vi "Cache.Result.Move.vi"(6 "Time (now)":timestamp, 8 "error in":errorcluster, 11 "File":path) -> (0 "error out":errorcluster)   [LabVIEW 2016]
uses:
  Global/ApplicationGlobal.vi
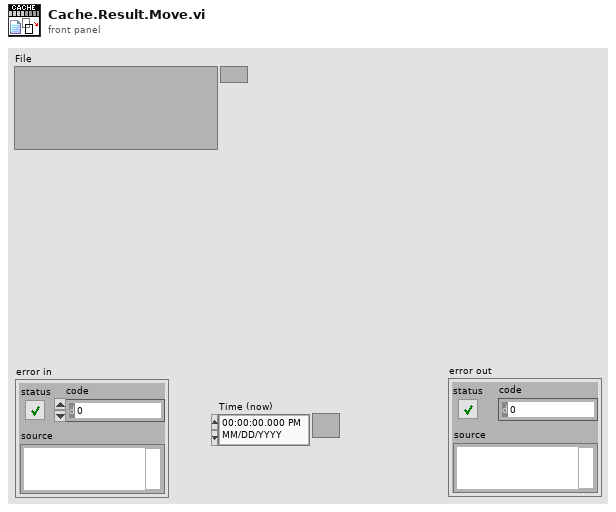
[diagram p1: front panel]
types:
  T1 = enum16{"open", "open or create", "create or replace", "create", "open (read-only)"}
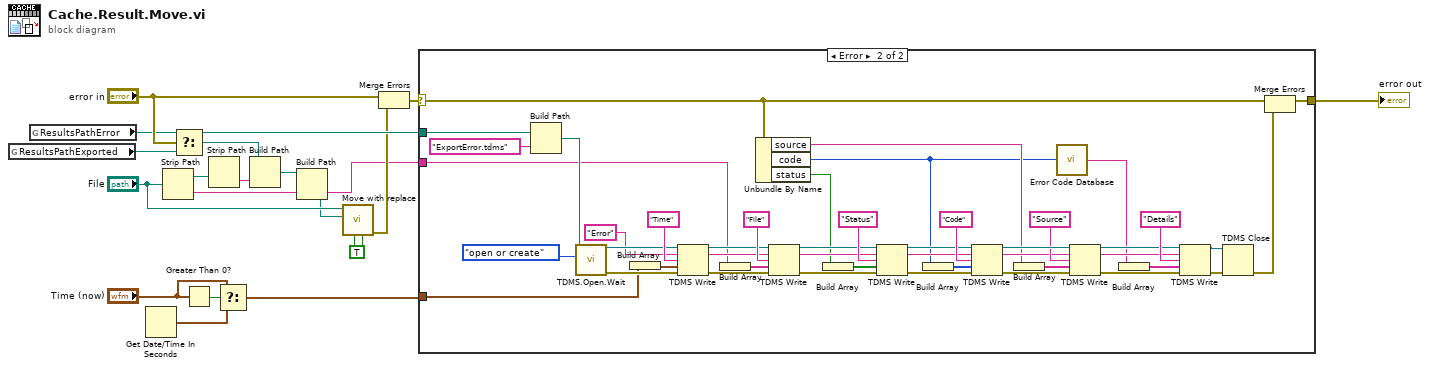
[diagram p0: block diagram]
diagram:
  w1 = TRUE ("create parent dirs (F)")
  n1 = global read "ApplicationGlobal.vi" "ResultsPathExported"() -> (w18:path)
  n2 = global read "ApplicationGlobal.vi" "ResultsPathError"() -> (w16:path)
  n3 = Get Date/Time In Seconds() -> (seconds since 1Jan1904=w12:timestamp)
  n4 = Strip Path(path="File") -> (stripped path=w4:path, name=w6:string)
  n5 = Select(t=w16, s="error in", f=w18) -> (s? t:f=w5:path)
  n6 = Greater Than 0?(x="Time (now)") -> (x > 0?=w13:bool)
  n7 = Strip Path(path=w4) -> (name=w3:string)  [unwired: 1 out]
  n8 = Select(t="Time (now)", s=w13, f=w12) -> (s? t:f=w10:timestamp)
  n9 = Build Path(base path=w5, name or relative path=w3) -> (appended path=w2:path)
  n10 = Build Path(base path=w2, name or relative path=w6) -> (appended path=w8:path)
  n11 = call "Move with replace.vi"("create parent dirs (F)"=w1, "replace allowed (T)"=w1, "destination path"=w8, "source path"="File") -> ("error"=w7:errorcluster)  [unwired: 7 in]
  n12 = Merge Errors("error in", w7) -> (w15:errorcluster)
  n13 = case shown="Error" w15 {
    selector: w15 -> [w19 w22]
    tunnel: w6 -> [_ w30]
    tunnel: w10 -> [_ w20]
    tunnel: w16 -> [_ w52]
    tunnel: [w19 w23] -> w14
    frame No Error {
    }
    frame Error {
      n14 = Build Path(base path=w52, name or relative path="ExportError.tdms") -> (appended path=w50:path)
      n15 = call "TDMS.Open.Wait.vi"("operation (open read-only)"=T1."open or create", "file path"=w50) -> ("error out"=w44:errorcluster, "tdms file out"=w47:refnum<k34>)  [unwired: 8 in]
      n16 = Build Array(w20) -> (w43:timestamp[])
      n17 = TDMS Write(0:w47, 5:"Error" ("group name in (Untitled)"), 7:"Time" ("channel name"), 9:w43, 11:w44) -> (4:w46:refnum<k34>, 6:w37:string, 15:w45:errorcluster)  [unwired: 1 in, 1 out]
      n18 = Build Array(w30) -> (w42:string[])
      n19 = Unbundle By Name(w22) -> ("source"=w28:string, "code"=w27:i32, "status"=w29:bool)
      n20 = TDMS Write(0:w46, 5:w37, 7:"File" ("channel name"), 9:w42, 11:w45) -> (4:w53:refnum<k34>, 6:w40:string, 15:w49:errorcluster)  [unwired: 1 in, 1 out]
      n21 = Build Array(w29) -> (w63:bool[])
      n22 = TDMS Write(0:w53, 5:w40, 7:"Status" ("channel name"), 9:w63, 11:w49) -> (4:w60:refnum<k34>, 6:w39:string, 15:w59:errorcluster)  [unwired: 1 in, 1 out]
      n23 = Build Array(w27) -> (w58:i32[])
      n24 = TDMS Write(0:w60, 5:w39, 7:"Code" ("channel name"), 9:w58, 11:w59) -> (4:w57:refnum<k34>, 6:w38:string, 15:w56:errorcluster)  [unwired: 1 in, 1 out]
      n25 = Build Array(w28) -> (w41:string[])
      n26 = call <vilib>:"Error Code Database.vi"("Error Code"=w27) -> ("Error Text"=w25:string)
      n27 = TDMS Write(0:w57, 5:w38, 7:"Source" ("channel name"), 9:w41, 11:w56) -> (4:w33:refnum<k34>, 6:w31:string, 15:w32:errorcluster)  [unwired: 1 in, 1 out]
      n28 = Build Array(w25) -> (w26:string[])
      n29 = TDMS Write(0:w33, 5:w31, 7:"Details" ("channel name"), 9:w26, 11:w32) -> (4:w34:refnum<k34>, 15:w35:errorcluster)  [unwired: 1 in, 2 out]
      n30 = TDMS Close(8:w35, 11:w34) -> (0:w24:errorcluster)  [unwired: 1 out]
      n31 = Merge Errors(w22, w24) -> (w23:errorcluster)
    }
  }
  "error out" <- w14
